vi "GetLoadedProgram.vi"(0 "DashboardServer in":refnum<class "Dashboard Server.lvclass">, 5 "error in (no error)":errorcluster) -> (14 "DashboardServer out":refnum<class "Dashboard Server.lvclass">, 15 "loadedProgram":string, 19 "error out":errorcluster)   [LabVIEW 2016, in "Dashboard Server.lvclass"]
uses:
  Dashboard Server.lvclass
panel:
  out "returnStatus":string
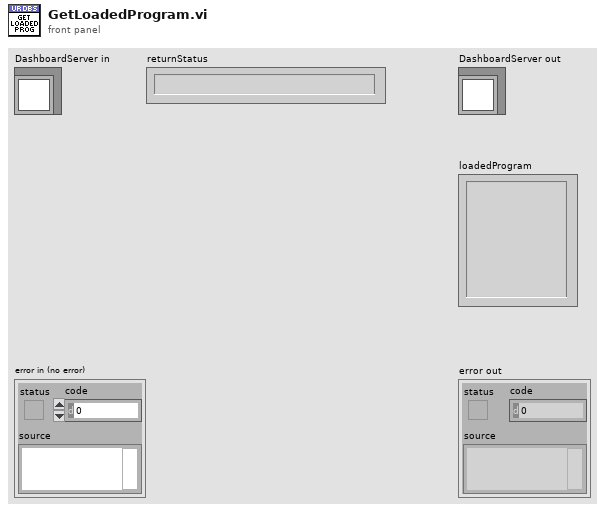
[diagram p1: front panel]
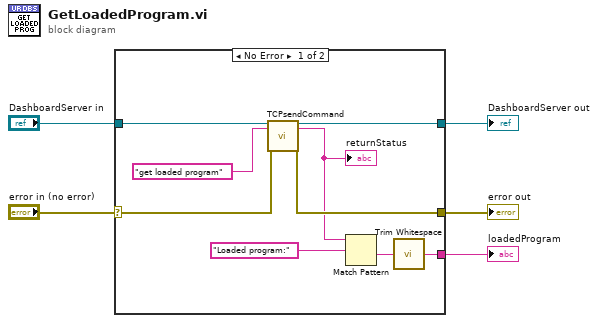
[diagram p0: block diagram]
diagram:
  n1 = case shown="No Error" "error in (no error)" {
    selector: "error in (no error)" -> [w12 w16]
    tunnel: [w11 w16] -> w4
    tunnel: [w13 w15] -> w2
    tunnel: "DashboardServer in" -> [w14 w15]
    tunnel: [w9 _] -> w1
    frame No Error {
      n2 = call-dynamic "TCPsendCommand.vi"("DashboardServer in"=w14, "command"="get loaded program", "error in (no error)"=w12) -> ("DashboardServer out"=w13:refnum<class "Dashboard Server.lvclass">, "returnStatus"=w8:string, "error out"=w11:errorcluster)  [unwired: 13 in, 1 out]
      "returnStatus" <- w8
      n3 = Match Pattern(string=w8, regular expression="Loaded program:") -> (after substring=w7:string)  [unwired: 1 in, 3 out]
      n4 = call <vilib>:"Trim Whitespace.vi"("string"=w7) -> ("trimmed string"=w9:string)  [unwired: 1 in]
    }
    frame Error {
    }
  }
  "error out" <- w4
  "DashboardServer out" <- w2
  "loadedProgram" <- w1
